vi "Path.vi"(10 "File":path, 11 "name or relative path":string) -> (3 "appended path":path)   [LabVIEW 2014]
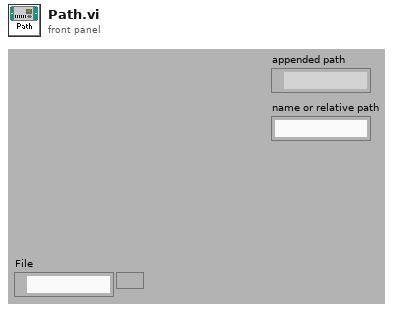
[diagram p1: front panel]
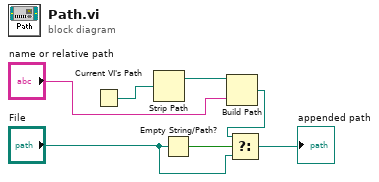
[diagram p0: block diagram]
diagram:
  n1 = Current VI's Path() -> (path=w7:path)
  n2 = Strip Path(path=w7) -> (stripped path=w6:path)  [unwired: 1 out]
  n3 = Empty String/Path?(string/path="File") -> (empty?=w3:bool)
  n4 = Build Path(base path=w6, name or relative path="name or relative path") -> (appended path=w2:path)
  n5 = Select(t=w2, s=w3, f="File") -> (s? t:f=→"appended path":path)
